vi "CustomErrors_NIcard.vi"(8 "error in (no error)":errorcluster) -> (0 "error out":errorcluster)   [LabVIEW 2013]
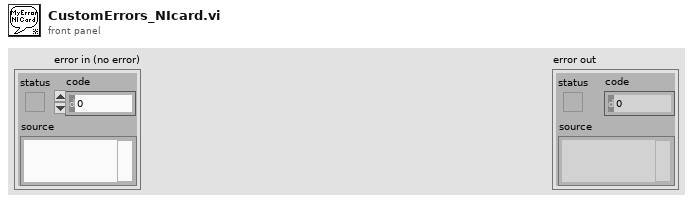
[diagram p1: front panel]
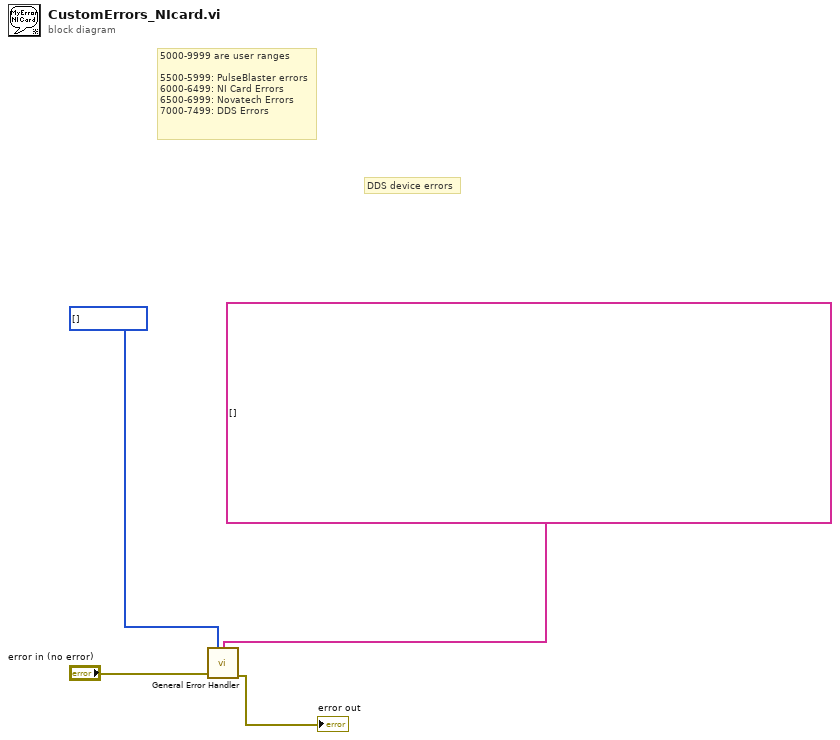
[diagram p0: block diagram]
diagram:
  # "DDS device errors"
  # "5000-9999 are user ranges\n\n5500-5999: PulseBlaster errors\n6000-6499: NI Card Errors\n6500-6999: Novatech Errors\n7000-7499: DDS Errors"
  n1 = call <vilib>:"General Error Handler.vi"("[user-defined codes]"=i32[] [], "[user-defined descriptions]"=string[] [], "error in (no error)"="error in (no error)") -> ("error out"=→"error out":errorcluster)  [unwired: 8 in, 4 out]
